vi "Data Logger Example.vi"(3 "2D Array":string[][](array[string])=[["Pin_Voltage", "Pin_Current", "Warning"], ["1", "0.1", "Very Low , Check"], ["2", "0.2", ""], ["3", "0.5", ""], ["4", "0.7", ""], ["5", "0.9", ""]], 8 "error in":errorcluster, 11 "Test Cluster":T1={"Numeric"=5.0, "String"="Test !", "Boolean"=FALSE, "Combo Box"="Combo 1", "Enum"=enum."Enum A", "Ring"=0, "Path"=path "C:/Path", "Array Of Digital"=[1.0, 2.0, 3.0], "Array Of String"=["Test 1", "Test 2", "Test 3"], "Array Of Boolean"=[FALSE, TRUE], "Array Of Ring"=[1, 0, 2]} {"Array Of Ring" items=["Ring 1", "Ring 2", "Ring 3"]; "Ring" items=["Ring 1", "Ring 2", "Ring 3"]}) -> (0 "error out":errorcluster)   [LabVIEW 2024, in "dataLogger.lvlib"]
uses:
  dataLogger.lvlib
panel:
  # "Data Logger Example"
  # "Run this VI and view the generated log file in the path: \n\nC:\\Users\\Public\\Documents\\National Instruments\\Test"
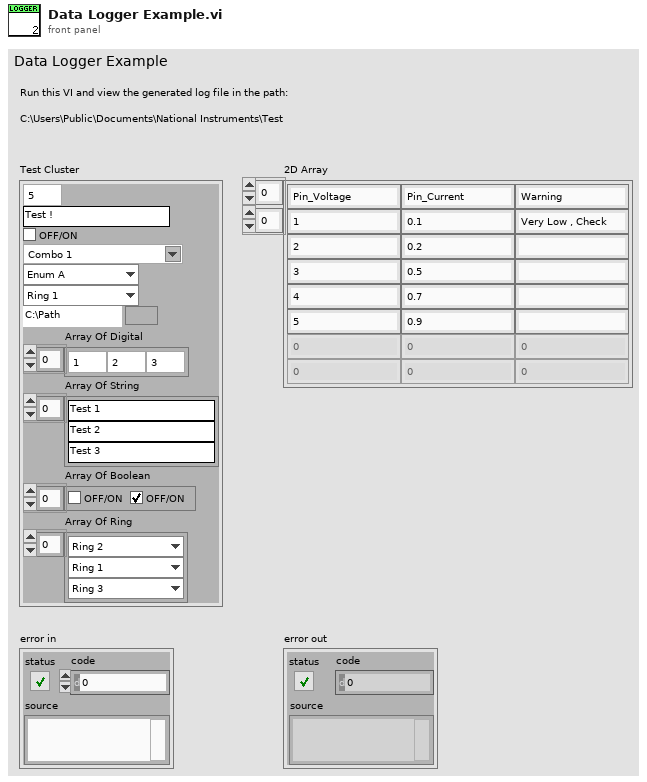
[diagram p1: front panel]
types:
  T1 = cluster{"Numeric":dbl, "String":string, "Boolean":bool, "Combo Box":string, "Enum":enum16{"Enum A", "Enum B", "Enum C"}, "Ring":u16, "Path":path, "Array Of Digital":dbl[], "Array Of String":string[], "Array Of Boolean":bool[], "Array Of Ring":u16[]}
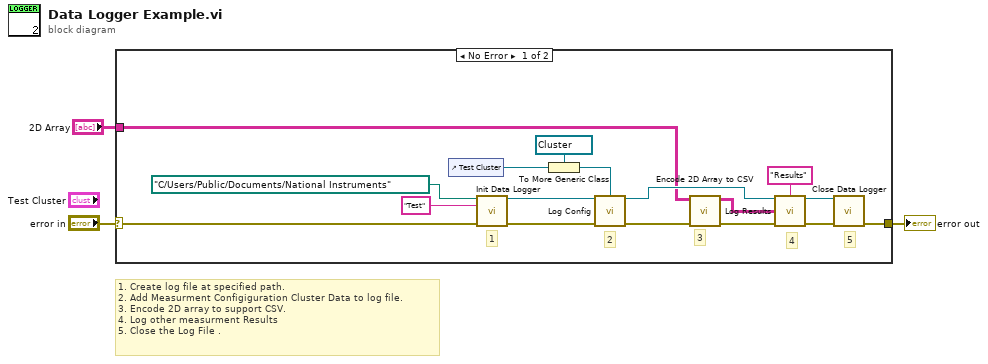
[diagram p0: block diagram]
diagram:
  # "1. Create log file at specified path.\n2. Add Measurment Configiguration Cluster Data to log file.\n3. Encode 2D array to support CSV.\n4. Log other measurment Results\n5. Close the Log File ."
  n1 = case shown="No Error" "error in" {
    selector: "error in" -> [w16 w21]
    tunnel: [w9 w21] -> w3
    tunnel: "2D Array" -> [w5 _]
    frame No Error {
      # "3"
      # "5"
      # "4"
      # "2"
      # "1"
      n2 = control-ref of="Test Cluster"() -> (w15:refnum<vi>)
      n3 = call "Init Data Logger.vi"("Log File Path"=path "C:/Users/Public/Documents/National Instruments" ("Log Path"), "Module"="Test" ("Service"), "error in"=w16) -> ("Log File Ref. Out"=w14:refnum<file>, "error out"=w19:errorcluster)  [unwired: 10 in, 1 out]
      n4 = To More Generic Class(target class=refnum<vi> refnum ("Measurement Config"), reference=w15) -> (generic class reference=w13:refnum<vi>)
      n5 = call "Log Config.vi"("Log File Ref In"=w14, "Measurement Config Ref."=w13, "error in"=w19) -> ("Log File Ref Out"=w12:refnum<file>, "error out"=w7:errorcluster)  [unwired: 10 in, 1 out]
      n6 = call "Encode 2D Array to CSV.vi"("error in"=w7, "2D Array In"=w5) -> ("error out"=w6:errorcluster, "2D Array Out"=w4:string[][])  [unwired: 8 in]
      n7 = call "Log Results.vi"("Log File Ref. In"=w12, "Results Name"="Results", "Data Input"=w4, "error in"=w6) -> ("Log File Ref. Out"=w8:refnum<file>, "error out"=w10:errorcluster)  [unwired: 9 in, 1 out]
      n8 = call "Close Data Logger.vi"("error in"=w10, "Log FIle Ref. In"=w8) -> ("error out"=w9:errorcluster)  [unwired: 9 in]
    }
    frame Error {
    }
  }
  "error out" <- w3
